vi "CV2PKdll.vi"(8 "error in (no error)":errorcluster, 11 "Inputs":cluster{"icomp":i32, "t":dbl, "D":dbl}) -> (0 "error out":errorcluster, 3 "Outputs":T1)   [LabVIEW 2021]
doc: "subroutine CV2PKdll(icomp, t, d, cv2p, csat, ierr, herr, herr_length)\n\nCompute the isochoric heat capacity in the two phase (liquid+vapor) region.\n\nINPUTS:\nicomp -- Component number in mixture (1..nc); 1 for pure fluid\nt -- Temperature [K]\nD -- Density [mol/L] if known If D=0, then a saturated liquid state is assumed.\n\nOUTPUTS:\ncv2p -- Isochoric two-phase heat capacity [J/mol-K]\ncsat -- Saturation heat capacity [J/mol-K] (Although there is already a Csat \n routine in REFPROP, it is also returned here. However, the calculation speed \n is slower than Csat.)\nierr -- error flag: 0 = successful\nherr -- error string \nherr_length -- length of variable herr (default: 255)"
uses:
  REFPROP.dll
panel:
  # "REFPROP-CV2PKdll.vi"
  # "void  CV2PKdll(int32_t *icomp, double *t, double *D, double *cv2p, double *csat, int32_t *ierr, CStr herr, int32_t herr_length)"
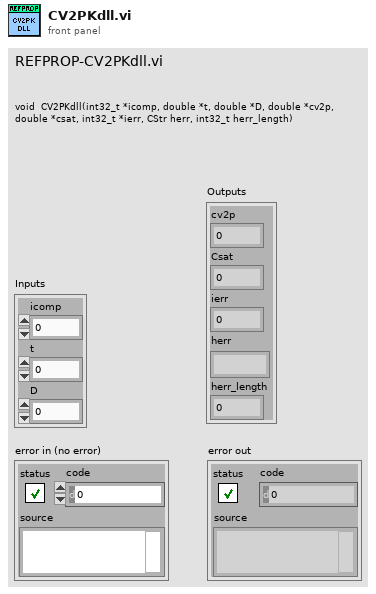
[diagram p1: front panel]
types:
  T1 = cluster{"cv2p":dbl, "Csat":dbl, "ierr":i32, "herr":string, "herr_length":i32}
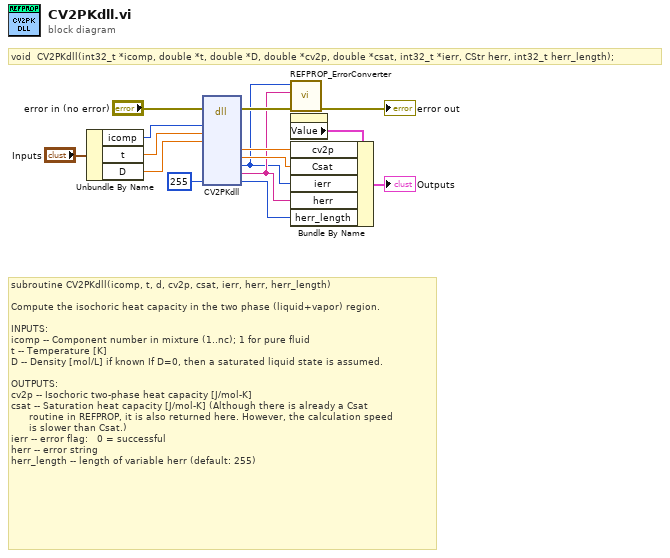
[diagram p0: block diagram]
diagram:
  # "void  CV2PKdll(int32_t *icomp, double *t, double *D, double *cv2p, double *csat, int32_t *ierr, CStr herr, int32_t herr_length);"
  # "subroutine CV2PKdll(icomp, t, d, cv2p, csat, ierr, herr, herr_length)\n\nCompute the isochoric heat capacity in the two phase (liquid+vapor) region.\n\nINPUTS:\nicomp -- Component number in mixture (1..nc); 1 for pure fluid\nt -- Temperature [K]\nD -- Density [mol/L] if known If D=0, then a saturated liquid state is assumed.\n\nOUTPUTS:\ncv2p -- Isochoric two-phase heat capacity [J/mol-K]\ncsat -- Saturation heat capacity [J/mol-K] (Although there is already a Csat    \n      routine in REFPROP, it is also returned here. However, the calculation speed \n      is slower than Csat.)\nierr -- error flag:   0 = successful\nherr -- error string \nherr_length -- length of variable herr (default: 255)"
  n1 = Unbundle By Name("Inputs") -> ("icomp"=w8:i32, "t"=w9:dbl, "D"=w10:dbl)
  n2 = dll-call lib="C:/Users/lauria/OneDrive - National Institute of Standards and Technology (NIST)/LabVIEW Projects/7 REFPROP/REFPROP-wrappers-master/REFPROP-wrappers-master/wrappers/Labview/REFPROP/REFPROP.*" fn="CV2PKdll"(error in="error in (no error)", "icomp"=w8, "t"=w9, "D"=w10, "herr_length"=255) -> (error out=w14:errorcluster, "cv2p"=w3:dbl, "csat"=w4:dbl, "ierr"=w1:i32, "herr"=w2:string, "herr_length"=w5:i32)  [unwired: 10 in, 1 out]
  n3 = call "REFPROP_ErrorConverter.vi"("error in (no error)"=w14, "Error Message"=w2, "Error Code"=w1) -> ("error out"=→"error out":errorcluster)  [unwired: 8 in]
  n4 = property on="Outputs" class="Clust (strict)"() -> ("Value"=w6:T1)  [unwired: 2 in, 2 out]
  n5 = Bundle By Name(cluster=w6, "cv2p"=w3, "Csat"=w4, "ierr"=w1, "herr"=w2, "herr_length"=w5) -> (→"Outputs":T1)
